vi "Handle Script Reply Payload as Cluster.vi"(8 "Action":enum16{"Read", "Write", "Delete"}(ring), 11 "Script Payload as Cluster in":bool) -> (3 "Script Payload as Cluster":bool)   [LabVIEW 2020, in "Panther Dashboard.lvlib"]
doc: "The intention of this VI is to\nEnable/Disable Panther Dashboard\nUIS, when Disabled, the Default\nDQMH UIs will be Used"
uses:
  Panther Dashboard.lvlib
  <resource>/dialog/lvconfig.llb/LV Config Read Boolean.vi
  <resource>/dialog/lvconfig.llb/LV Config Write Boolean.vi
panel:
  out "error out":errorcluster
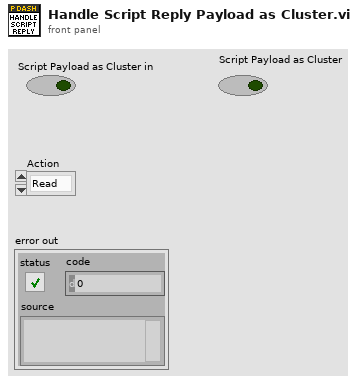
[diagram p1: front panel]
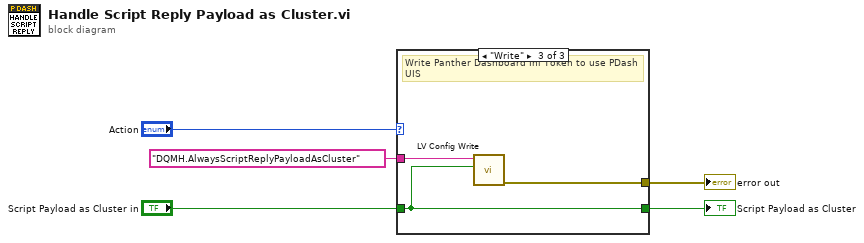
[diagram p0: block diagram]
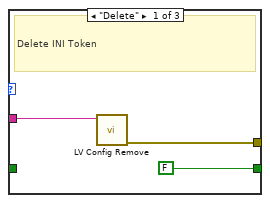
[diagram p2: hidden frame]
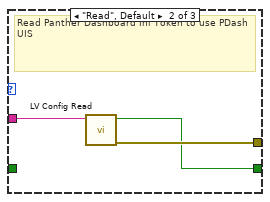
[diagram p3: hidden frame]
diagram:
  n1 = case shown="\"Write\"" "Action" {
    tunnel: "DQMH.AlwaysScriptReplyPayloadAsCluster" ("key") -> [w7 w10 w13]
    tunnel: [FALSE ("found?") w9 w12] -> w3
    tunnel: [w8 w11 w14] -> w5
    tunnel: "Script Payload as Cluster in" -> [_ _ w12]
    frame "Delete" {
      # "Delete INI Token"
      n2 = call <resource>:"LV Config Remove.vi"("key"=w7) -> ("error out"=w8:errorcluster)  [unwired: 6 in]
    }
    frame "Read", Default {
      # "Read Panther Dashboard Ini Token to use PDash UIS"
      n3 = call-poly <resource>:"LV Config Read.vi"("key"=w10) -> ("error out"=w11:errorcluster, "value"=w9:bool)  [unwired: 4 in, 1 out]
    }
    frame "Write" {
      # "Write Panther Dashboard Ini Token to use PDash UIS"
      n4 = call-poly <resource>:"LV Config Write.vi"("value"=w12, "key"=w13) -> ("error out"=w14:errorcluster)  [unwired: 5 in]
    }
  }
  "Script Payload as Cluster" <- w3
  "error out" <- w5
